vi "Think.vi"(6 "Target":i32, 7 "Target Locations":i32[][](array[numeric]), 9 "Current Heading":i32, 10 "dhead":i32) -> (2 "Executable Primitive":string, 4 "Desired Y":i32, 5 "Desired X":i32)   [LabVIEW 2012]
uses:
  <vilib>/imath/engines/lvmath/Plug In/_Char/NIMS_CH_character datatype.ctl
  <vilib>/imath/engines/lvmath2/RunTimeEngine/ErrorHandling/NIMS_Finalize Error.vi
  <vilib>/imath/engines/lvmath2/RunTimeEngine/Managers/WorkSpace/UID Generator.vi
  <vilib>/imath/engines/lvmath2/RunTimeEngine/Managers/SymbolTable/Clear UID.vi
  <vilib>/imath/engines/lvmath/Plug In/_Char/NIMS_CH_Character RV to String.vi
  <vilib>/imath/engines/lvmath2/RunTimeEngine/NodeEndStatement/NIMS_NodeEndStatement_Output.vi
  <instcachedir>/0/NIMS_NodeEndStatement_Output_53EC0D466D134D7ABD903AC30B43404B.lvgen/NIMS_NodeEndStatement_Output_53EC0D466D134D7ABD903AC30B43404B_009.vi
  <vilib>/imath/engines/lvmath2/RunTimeEngine/BuiltInFunctions/mod/NIMS_mod_no_size_check.vi
  <instcachedir>/0/NIMS_mod_no_size_check_5393E3382FD241D281EEB71DA286C65B.lvgen/NIMS_mod_no_size_check_5393E3382FD241D281EEB71DA286C65B_008.vi
  <vilib>/imath/engines/lvmath2/RunTimeEngine/RunTimeType/NIMS_RunTimeType_From StrictType (excl LVString).vi
  <instcachedir>/0/NIMS_RunTimeType_From StrictType (excl LVString)_AC52D965D0864706932D20A05968E122.lvgen/NIMS_RunTimeType_From StrictType (excl LVString)_AC52D965D0864706932D20A05968E122_001.vi
  <vilib>/imath/engines/lvmath2/RunTimeEngine/LocalVariableDefStatement/MC_LocalVariableDefStatement_Display.vi
  <vilib>/imath/engines/lvmath2/RunTimeEngine/Managers/SymbolTable/NIMS_WorkSpace.lvlib
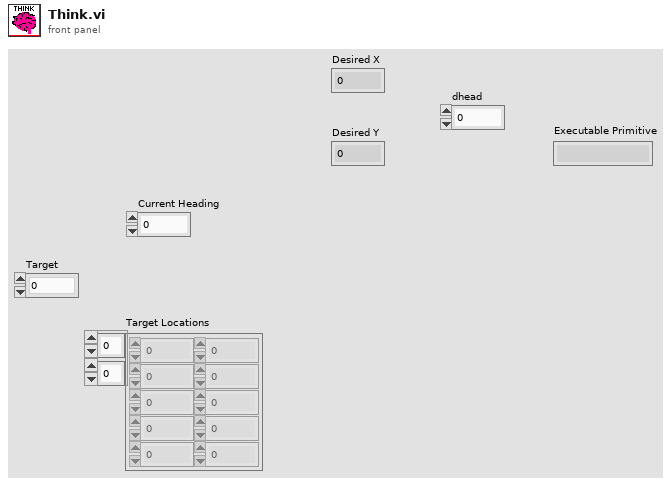
[diagram p1: front panel]
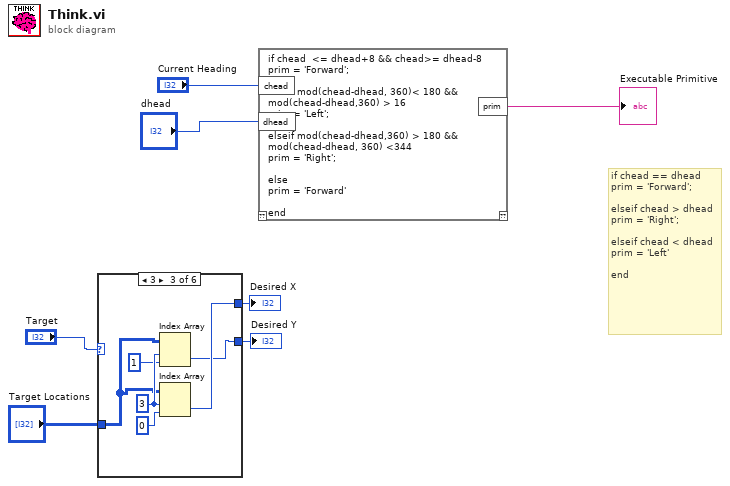
[diagram p0: block diagram]
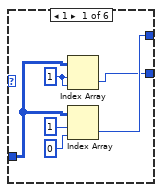
[diagram p2: hidden frame]
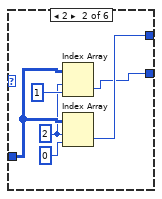
[diagram p3: hidden frame]
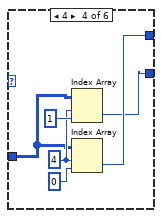
[diagram p4: hidden frame]
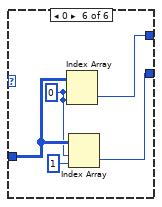
[diagram p6: hidden frame]
diagram:
  # "if chead == dhead\nprim = 'Forward';\n\nelseif chead > dhead\nprim = 'Right';\n\nelseif chead < dhead\nprim = 'Left'\n\nend"
  n1 = case shown="3" "Target" {
    tunnel: "Target Locations" -> [w12 w15 w20 w26 _ w35]
    tunnel: [w11 w17 w22 w28 _ w36] -> w4
    tunnel: [w10 w16 w21 w27 _ w32] -> w5
    frame 1 {
      w8 = 1 ("disabled index (col)")
      n2 = Index Array(array=w12, index (row)=w8, index (col)=w8) -> (element=w10:i32)
      n3 = Index Array(array=w12, index (row)=1, index (col)=0 ("disabled index (col)")) -> (element=w11:i32)
    }
    frame 2 {
      w14 = 2 ("index (row)")
      n4 = Index Array(array=w15, index (row)=w14, index (col)=1 ("disabled index (col)")) -> (element=w16:i32)
      n5 = Index Array(array=w15, index (row)=w14, index (col)=0 ("disabled index (col)")) -> (element=w17:i32)
    }
    frame 3 {
      w25 = 3 ("index (row)")
      n6 = Index Array(array=w20, index (row)=w25, index (col)=1 ("disabled index (col)")) -> (element=w21:i32)
      n7 = Index Array(array=w20, index (row)=w25, index (col)=0 ("disabled index (col)")) -> (element=w22:i32)
    }
    frame 4 {
      w29 = 4 ("index (row)")
      n8 = Index Array(array=w26, index (row)=w29, index (col)=1 ("disabled index (col)")) -> (element=w27:i32)
      n9 = Index Array(array=w26, index (row)=w29, index (col)=0 ("disabled index (col)")) -> (element=w28:i32)
    }
    frame 5, Default {
    }
    frame 0 {
      w34 = 0 ("index (row)")
      n10 = Index Array(array=w35, index (row)=w34, index (col)=w34) -> (element=w36:i32)
      n11 = Index Array(array=w35, index (row)=w34, index (col)=1 ("disabled index (col)")) -> (element=w32:i32)
    }
  }
  "Desired X" <- w4
  "Desired Y" <- w5
  n12 = mathscript code="if chead  <= dhead+8 && chead>= dhead-8\nprim = 'Forward';\n\nelseif mod(chead-dhead, 360)< 180 && mod(chead-dhead,360) > 16\nprim = 'Left';\n\nelseif mod(chead-dhead,360) > 180 && mod(chead-dhead, 360) <344\nprim = 'Right';\n\nelse\nprim = 'Forward'\n\nend"("chead"="Current Heading", "dhead"="dhead") -> ("prim"=→"Executable Primitive":string)  [unwired: 1 in, 1 out]
